vi "createSetupXmlElement.vi"(8 "error in (no error)":errorcluster, 9 "Comment":string, 10 "Test ref":refnum<k20>, 11 "DOM document":refnum<k20>) -> (0 "error out":errorcluster, 1 "Setup ref":refnum<k20>, 2 "dup Test ref":refnum<k20>, 3 "dup DOM document":refnum<k20>)   [LabVIEW 2013]
uses:
  <resource>/objmgr/DOMUserDefRef.rc
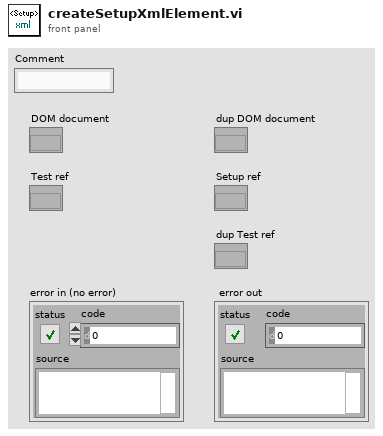
[diagram p1: front panel]
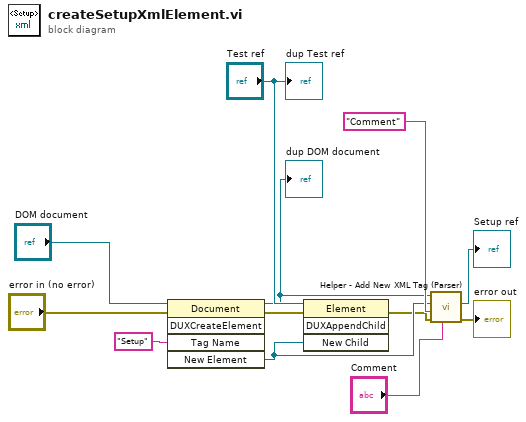
[diagram p0: block diagram]
diagram:
  n1 = invoke class="Document" method="DUXCreateElement"(reference="DOM document", error in="error in (no error)", "Tag Name"="Setup" ("Qualified Name")) -> (reference out=w5:refnum<k20>, error out=w10:errorcluster, "New Element"=w6:refnum<k20>)  [unwired: 2 in, 2 out]
  "dup DOM document" <- w5
  n2 = invoke class="Element" method="DUXAppendChild"(reference="Test ref", error in=w10, "New Child"=w6) -> (error out=w3:errorcluster)  [unwired: 1 in, 3 out]
  n3 = call "Helper - Add New XML Tag (Parser).vi"("Tag Data"="Comment", "error in (no error)"=w3, "Tag Name"="Comment" ("Qualified Name"), "Owning Element"=w6, "DOM document"=w5) -> ("error out"=→"error out":errorcluster, "dup Owning Element"=→"Setup ref":refnum<k20>)  [unwired: 4 in, 1 out]
  "dup Test ref" <- "Test ref"
